vi "空载判定.vi"(0 "曲线引用":refnum<vi>, 1 "曲线":u32, 2 "曲线判定条件":T1, 3 "错误输入":errorcluster) -> (7 "曲线引用输出":refnum<vi>, 8 "判定结果":cluster{"合格？":bool, "判定结果":string[][]}, 10 "错误输出":errorcluster)   [LabVIEW 2018]
uses:
  <userlib>/_MGI/1D Array/MGI Average/MGI Average (DBL[]).vi
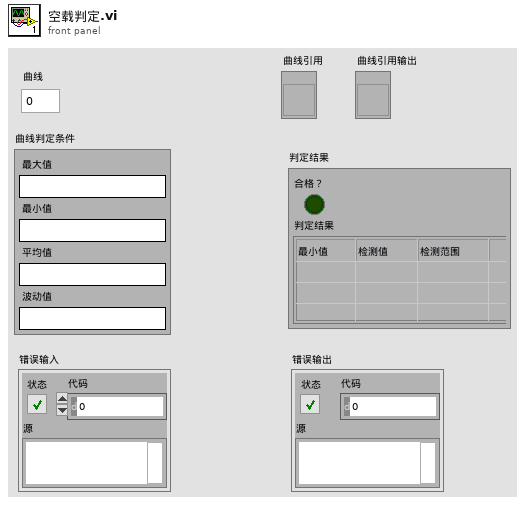
[diagram p1: front panel]
types:
  T1 = cluster{"最大值":string, "最小值":string, "平均值":string, "波动值":string}
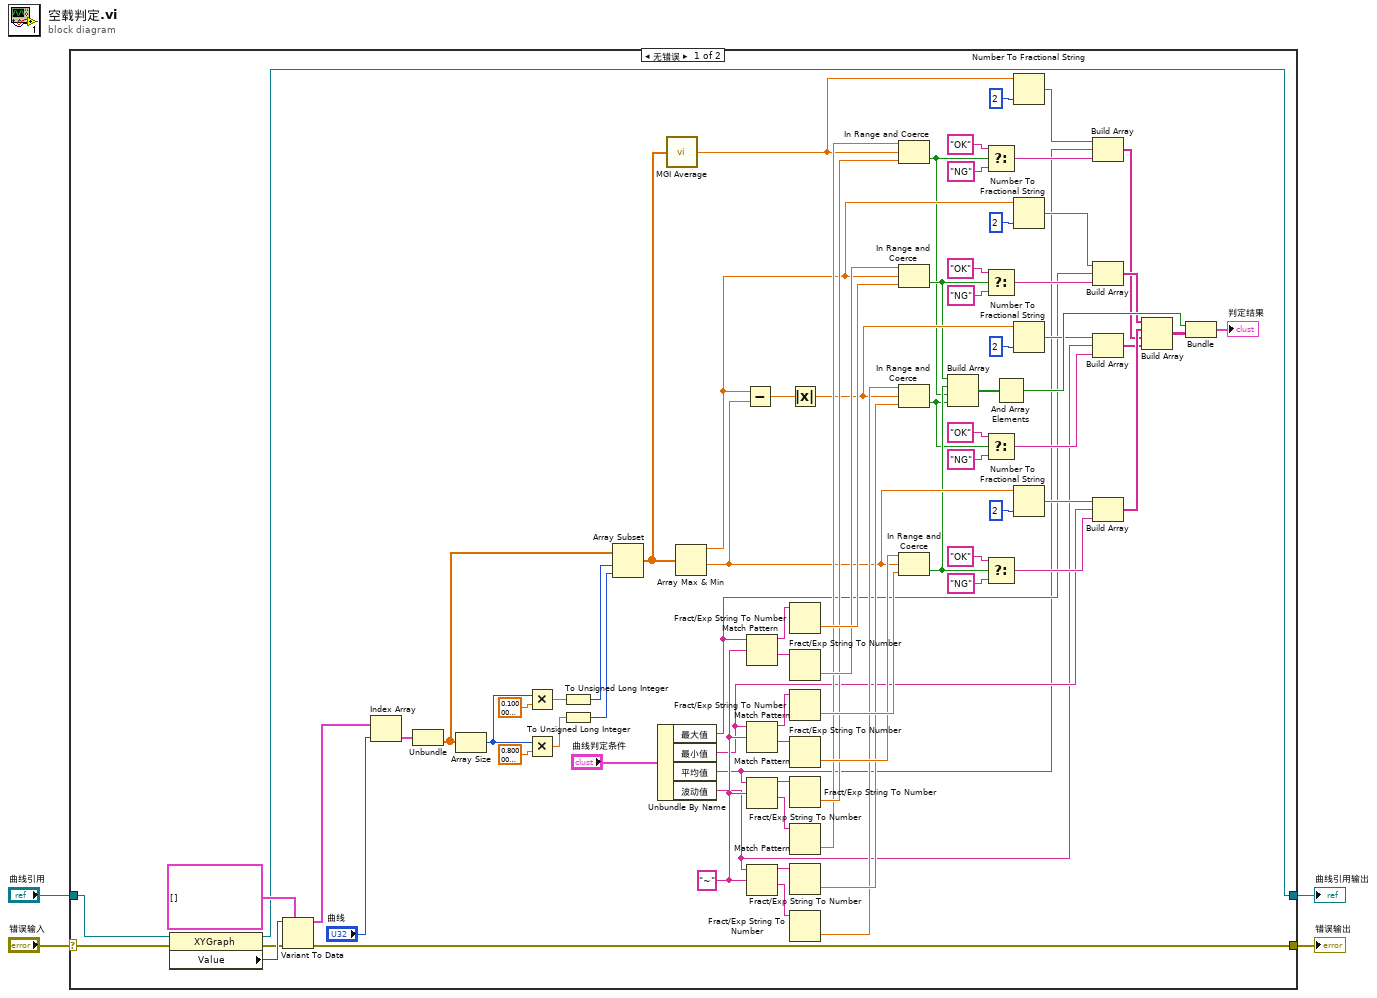
[diagram p0: block diagram]
diagram:
  n1 = case shown="无错误" "错误输入" {
    selector: "错误输入" -> [w80 w84]
    tunnel: [w41 w84] -> w3
    tunnel: "曲线引用" -> [w44 w83]
    tunnel: [w43 w83] -> w1
    frame No Error {
      w78 = "~" ("正则表达式")
      n2 = property class="XYGraph"(reference=w44, error in=w80) -> (reference out=w43:refnum<vi>, error out=w42:errorcluster, "Value"=w82:variant)
      n3 = Variant To Data(error in=w42, type=cluster{dbl[], dbl[]}[] [], Variant=w82) -> (data=w33:cluster{dbl[], dbl[]}[], error out=w41:errorcluster)
      n4 = Index Array(array=w33, index="曲线") -> (element=w77:cluster{dbl[], dbl[]})
      n5 = Unbundle(w77) -> (w32:dbl[])  [unwired: 1 out]
      n6 = Array Size(array=w32) -> (size(s)=w37:i32)
      n7 = Multiply(x=w37, y=sgl 0.1) -> (x*y=w36:sgl)
      n8 = Multiply(x=w37, y=sgl 0.8) -> (x*y=w38:sgl)
      n9 = To Unsigned Long Integer(number=w36) -> (unsigned 32bit integer=w39:u32)
      n10 = To Unsigned Long Integer(number=w38) -> (unsigned 32bit integer=w40:u32)
      n11 = Array Subset(array=w32, index=w39, length=w40) -> (w31:dbl[])
      n12 = Unbundle By Name("曲线判定条件") -> ("最大值"=w12:string, "最小值"=w11:string, "平均值"=w9:string, "波动值"=w10:string)
      n13 = call-poly <userlib>:"MGI Average.vi"("Double[]"=w31) -> ("Average"=w52:dbl)  [unwired: 1 in]
      n14 = Array Max & Min(array=w31) -> (max value=w56:dbl, min value=w58:dbl)  [unwired: 2 out]
      n15 = Subtract(x=w56, y=w58) -> (x-y=w59:dbl)
      n16 = Match Pattern(string=w12, regular expression=w78) -> (before substring=w75:string, after substring=w74:string)  [unwired: 1 in, 2 out]
      n17 = Match Pattern(string=w11, regular expression=w78) -> (before substring=w73:string, after substring=w72:string)  [unwired: 1 in, 2 out]
      n18 = Match Pattern(string=w9, regular expression=w78) -> (before substring=w71:string, after substring=w70:string)  [unwired: 1 in, 2 out]
      n19 = Match Pattern(string=w10, regular expression=w78) -> (before substring=w69:string, after substring=w68:string)  [unwired: 1 in, 2 out]
      n20 = Absolute Value(x=w59) -> (abs(x)=w51:dbl)
      n21 = Fract/Exp String To Number(string=w75) -> (number=w67:dbl)  [unwired: 3 in, 1 out]
      n22 = Fract/Exp String To Number(string=w74) -> (number=w66:dbl)  [unwired: 3 in, 1 out]
      n23 = Fract/Exp String To Number(string=w73) -> (number=w65:dbl)  [unwired: 3 in, 1 out]
      n24 = Fract/Exp String To Number(string=w72) -> (number=w64:dbl)  [unwired: 3 in, 1 out]
      n25 = Fract/Exp String To Number(string=w71) -> (number=w63:dbl)  [unwired: 3 in, 1 out]
      n26 = Fract/Exp String To Number(string=w70) -> (number=w62:dbl)  [unwired: 3 in, 1 out]
      n27 = Fract/Exp String To Number(string=w69) -> (number=w61:dbl)  [unwired: 3 in, 1 out]
      n28 = Fract/Exp String To Number(string=w68) -> (number=w60:dbl)  [unwired: 3 in, 1 out]
      n29 = In Range and Coerce(upper limit=w62, x=w52, lower limit=w63) -> (In Range?=w20:bool)  [unwired: 1 out]
      n30 = In Range and Coerce(upper limit=w66, x=w56, lower limit=w67) -> (In Range?=w24:bool)  [unwired: 1 out]
      n31 = In Range and Coerce(upper limit=w60, x=w51, lower limit=w61) -> (In Range?=w18:bool)  [unwired: 1 out]
      n32 = In Range and Coerce(upper limit=w64, x=w58, lower limit=w65) -> (In Range?=w22:bool)  [unwired: 1 out]
      n33 = Build Array(w24, w22, w20, w18) -> (w50:bool[])
      n34 = Select(t="OK", s=w20, f="NG") -> (s? t:f=w19:string)
      n35 = Select(t="OK", s=w24, f="NG") -> (s? t:f=w23:string)
      n36 = Select(t="OK", s=w18, f="NG") -> (s? t:f=w17:string)
      n37 = Select(t="OK", s=w22, f="NG") -> (s? t:f=w21:string)
      n38 = And Array Elements(Boolean array=w50) -> (logical AND=w47:bool)
      n39 = Number To Fractional String(number=w52, precision (6)=i16 2 ("精度(6)")) -> (F-format string=w15:string)  [unwired: 2 in]
      n40 = Number To Fractional String(number=w56, precision (6)=i16 2 ("精度(6)")) -> (F-format string=w13:string)  [unwired: 2 in]
      n41 = Number To Fractional String(number=w51, precision (6)=i16 2 ("精度(6)")) -> (F-format string=w16:string)  [unwired: 2 in]
      n42 = Number To Fractional String(number=w58, precision (6)=i16 2 ("精度(6)")) -> (F-format string=w14:string)  [unwired: 2 in]
      n43 = Build Array(w15, w9, w19) -> (w6:string[])
      n44 = Build Array(w13, w12, w23) -> (w8:string[])
      n45 = Build Array(w16, w10, w17) -> (w5:string[])
      n46 = Build Array(w14, w11, w21) -> (w7:string[])
      n47 = Build Array(w8, w7, w6, w5) -> (w45:string[][])
      n48 = Bundle(w47, w45) -> (→"判定结果":cluster{bool, string[][]})  [unwired: 1 in]
    }
    frame Error {
    }
  }
  "错误输出" <- w3
  "曲线引用输出" <- w1
